vi "potenciometro_gauge.vi"() -> ()   [LabVIEW 2018]
uses:
  <vilib>/Instr/_visa.llb/VISA Configure Serial Port (Instr).vi
panel:
  in  "stop":bool
  out "Gauge":dbl(knob) scale=0.0..1023.0
  in  "VISA resource name":refnum<visa-resource-name>
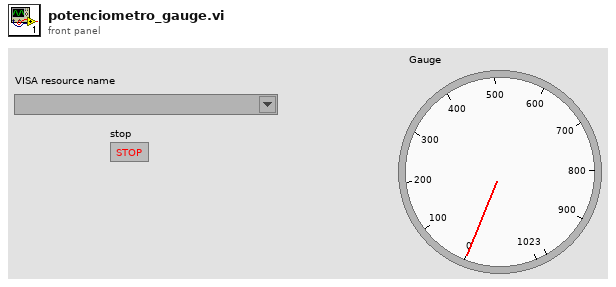
[diagram p1: front panel]
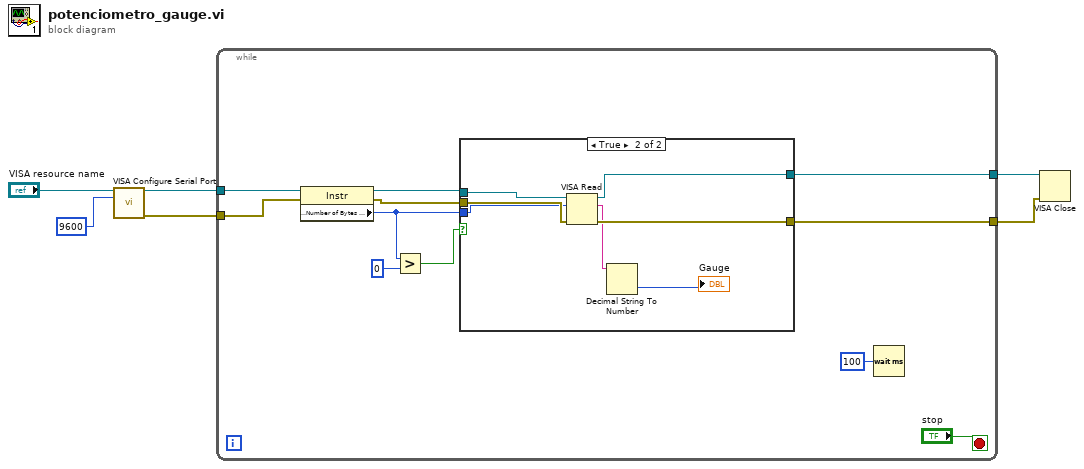
[diagram p0: block diagram]
diagram:
  n1 = call-poly "VISA Configure Serial Port"("VISA resource name"="VISA resource name", "baud rate (9600)"=u32 9600) -> ("VISA resource name out"=w4:refnum<visa-resource-name>, "error out"=w3:errorcluster)  [unwired: 12 in]
  n2 = while {
    tunnel: w4 -> [w17]
    tunnel: w3 -> [w16]
    tunnel: [w14] -> w2
    tunnel: [w13] -> w1
    stop <- "stop" stop-if-true
    n3 = property class="Instr"(reference=w17, error in=w16) -> (reference out=w10:refnum<visa-resource-name>, error out=w9:errorcluster, "Serial Settings:Number of Bytes at Serial Port"=w8:u32)
    n4 = Greater?(x=w8, y=u32 0) -> (0:w15:bool)
    n5 = case shown="True" w15 {
      tunnel: [w19 w25] -> w14
      tunnel: [w18 w24] -> w13
      tunnel: w10 -> [w19 w23]
      tunnel: w9 -> [w18 w22]
      tunnel: w8 -> [_ w21]
      frame False {
      }
      frame True {
        n6 = VISA Read(VISA resource name=w23, byte count=w21, error in (no error)=w22) -> (VISA resource name out=w25:refnum<visa-resource-name>, read buffer=w20:string, error out=w24:errorcluster)  [unwired: 1 out]
        n7 = Decimal String To Number(string=w20) -> (number=→"Gauge":i32)  [unwired: 2 in, 1 out]
      }
    }
    n8 = Wait (ms)(milliseconds to wait=u32 100) -> ()  [unwired: 1 out]
  }
  n9 = VISA Close(VISA resource name=w2, error in (no error)=w1) -> ()  [unwired: 1 out]
